vi "DualPower.vi"() -> ()   [LabVIEW 2019]
panel:
  in  "Numeric 2":dbl
  in  "Numeric":dbl
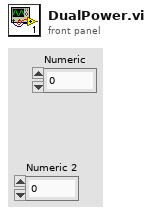
[diagram p1: front panel]
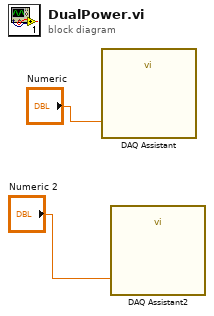
[diagram p0: block diagram]
diagram:
  n1 = call "DAQ Assistant"("data"="Numeric") -> ()  [unwired: 17 in, 2 out]
  n2 = call "DAQ Assistant2"("data"="Numeric 2") -> ()  [unwired: 17 in, 2 out]
